vi "Check Listener.vi"(8 "error in (no error)":errorcluster, 11 "Messaging Server Module in":refnum<class "Messaging Server Module.lvclass">) -> (0 "error out":errorcluster, 3 "Messaging Server Module out":refnum<class "Messaging Server Module.lvclass">)   [LabVIEW 2020, in "Volatus.lvlib" / "Messaging Server Module.lvclass"]
uses:
  Messaging Server Module.lvclass
  Messaging Server Module.lvclass/Messaging Server Module.ctl
  lv-vecto/Vecto/IP Resolver/IP Resolver.lvclass
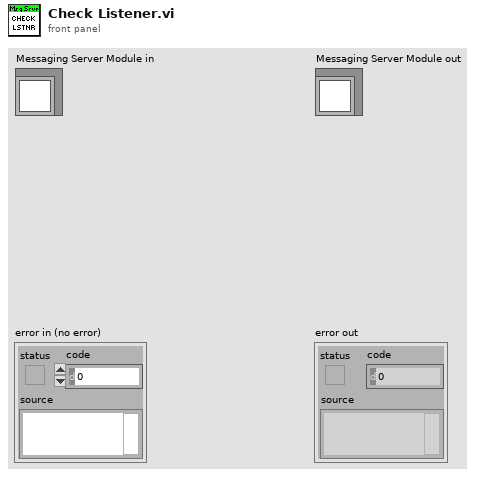
[diagram p1: front panel]
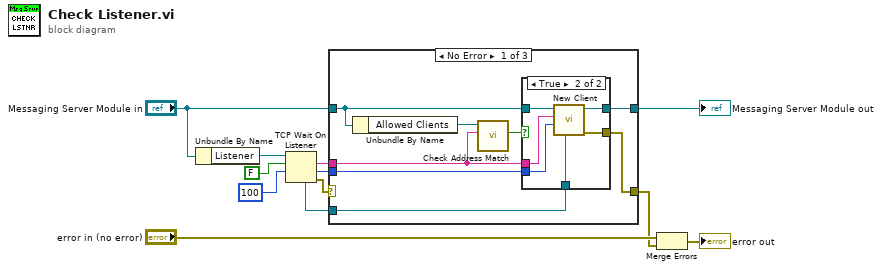
[diagram p0: block diagram]
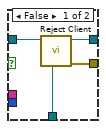
[diagram p2: hidden frame]
diagram:
  n1 = Unbundle By Name("Messaging Server Module in") -> ("Listener"=w11:refnum<k5>)
  n2 = TCP Wait On Listener(9:100 ("timeout ms (wait forever: -1)"), 10:FALSE ("resolve remote address (T)"), 11:w11) -> (0:w8:errorcluster, 1:w6:u16, 2:w5:string, 4:w7:refnum<k5>)  [unwired: 1 in, 1 out]
  n3 = case shown="No Error" w8 {
    selector: w8 -> [_ _ w32]
    tunnel: w7 -> [w19 _ _]
    tunnel: w6 -> [w20 _ _]
    tunnel: w5 -> [w14 _ _]
    tunnel: "Messaging Server Module in" -> [w16 w31 w33]
    tunnel: [w17 w31 w33] -> w3
    tunnel: [w18 _ w32] -> w1
    frame No Error {
      n4 = Unbundle By Name(w16) -> ("Allowed Clients"=w15:refnum<class "IP Resolver.lvclass">)
      n5 = call "Check Address Match.vi"("Address"=w14, "IP Resolver in"=w15) -> ("Matches"=w13:bool)  [unwired: 7 in, 2 out]
      n6 = case shown="True" w13 {
        tunnel: w20 -> [_ w30]
        tunnel: w19 -> [w22 w29]
        tunnel: [w21 w28] -> w18
        tunnel: [w23 w27] -> w17
        tunnel: w16 -> [w24 w26]
        tunnel: w14 -> [_ w25]
        frame False {
          n7 = call "Reject Client.vi"("Client"=w22, "Messaging Server Module in"=w24) -> ("error out"=w21:errorcluster, "Messaging Server Module out"=w23:refnum<class "Messaging Server Module.lvclass">)  [unwired: 8 in]
        }
        frame True {
          n8 = call "New Client.vi"("Client"=w29, "Port"=w30, "Address"=w25, "Messaging Server Module in"=w26) -> ("error out"=w28:errorcluster, "Messaging Server Module out"=w27:refnum<class "Messaging Server Module.lvclass">)  [unwired: 6 in]
        }
      }
    }
    frame Error {
      # "No new client, not actually an error."
    }
    frame Default {
    }
  }
  "Messaging Server Module out" <- w3
  n9 = Merge Errors("error in (no error)", w1) -> (→"error out":errorcluster)
